vi "XYStage_Write_General_Command.vi"(5 "Timeout":i32, 7 "Command Delay":i32, 8 "error in (no error)":errorcluster, 9 "Expected Reply":string, 10 "Command to Execute":string, 11 "VISA resource name":refnum<visa-resource-name>) -> (0 "error out":errorcluster, 2 "Stage Response":string, 3 "VISA resource name out":refnum<visa-resource-name>)   [LabVIEW 2013]
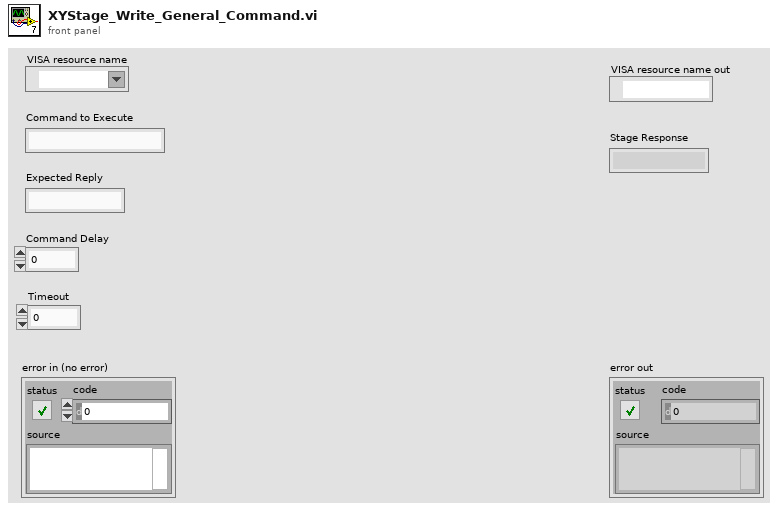
[diagram p1: front panel]
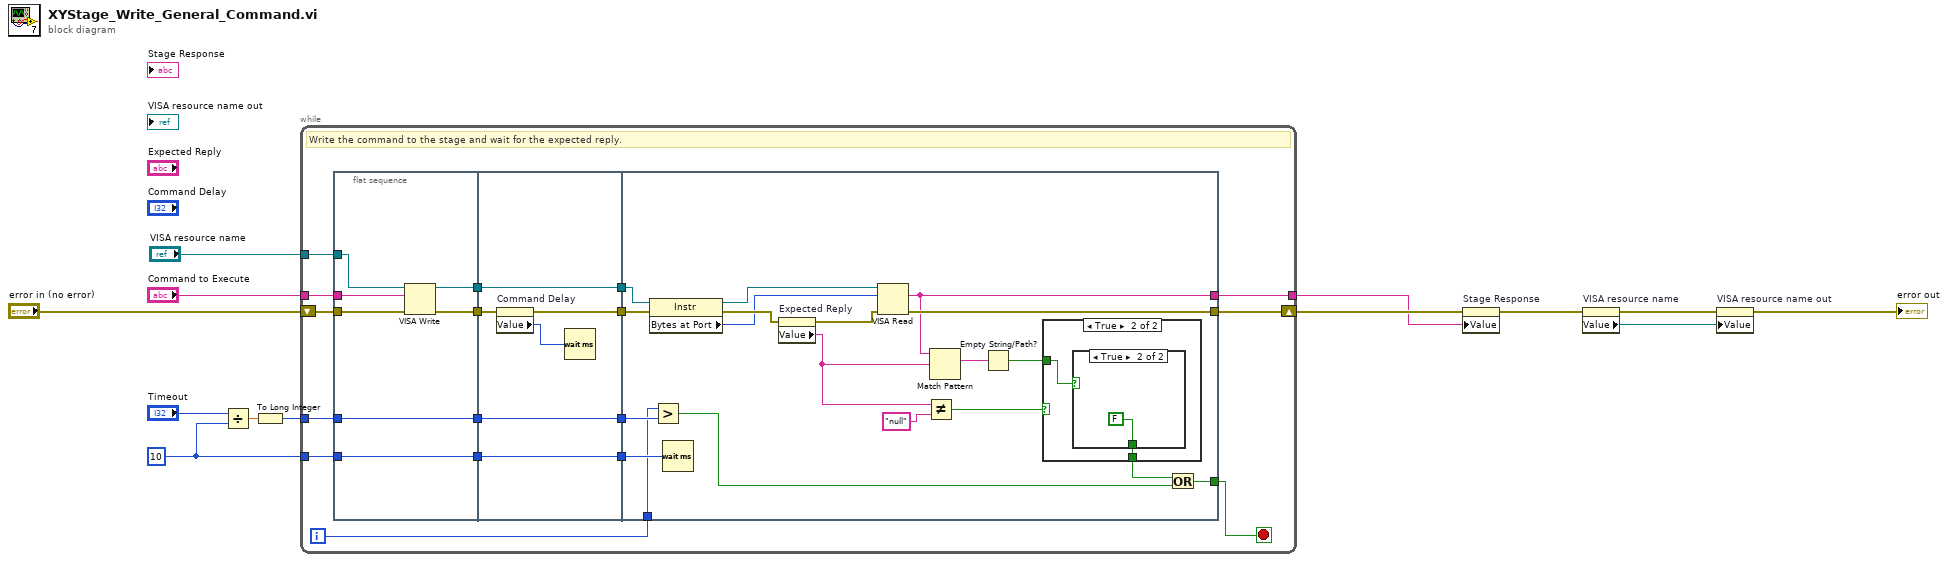
[diagram p0: block diagram]
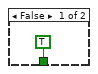
[diagram p2: hidden frame]
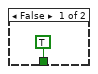
[diagram p3: hidden frame]
diagram:
  w9 = 10
  n1 = Divide(x="Timeout", y=w9) -> (x/y=w11:dbl)
  n2 = To Long Integer(number=w11) -> (32bit integer=w10:i32)
  n3 = while {
    tunnel: "VISA resource name" -> [w30]
    tunnel: "Command to Execute" -> [w29]
    shift-right: [w22] -> w6
    shift-left: "error in (no error)" -> [w28]
    tunnel: [w21] -> w5
    tunnel: w10 -> [w17]
    tunnel: w9 -> [w20]
    i -> [w14]
    stop <- w23 stop-if-true
    # "Write the command to the stage and wait for the expected reply."
    n4 = flat-sequence {
      tunnel: w30 -> [w37]
      tunnel: w29 -> [w36]
      tunnel: w28 -> [w35]
      tunnel: [w34] -> w27
      tunnel: [w33] -> w26
      tunnel: w20 -> [w32]
      tunnel: [w32] -> w19
      tunnel: w17 -> [w31]
      tunnel: [w31] -> w15
      tunnel: w27 -> [w40]
      tunnel: w26 -> [w43]
      tunnel: [w42] -> w25
      tunnel: [w40] -> w24
      tunnel: w19 -> [w39]
      tunnel: [w39] -> w18
      tunnel: [w38] -> w16
      tunnel: w15 -> [w38]
      tunnel: w25 -> [w62]
      tunnel: w24 -> [w61]
      tunnel: [w52] -> w23
      tunnel: w18 -> [w48]
      tunnel: w16 -> [w47]
      tunnel: w14 -> [w46]
      tunnel: [w50] -> w22
      tunnel: [w49] -> w21
      frame #0 {
        n5 = VISA Write(VISA resource name=w37, write buffer=w36, error in (no error)=w35) -> (VISA resource name out=w34:refnum<visa-resource-name>, error out=w33:errorcluster)  [unwired: 1 out]
      }
      frame #1 {
        n6 = property on="Command Delay" class="DigNum (strict)"(error in=w43) -> (error out=w42:errorcluster, "Value"=w41:i32)  [unwired: 1 in, 1 out]
        n7 = Wait (ms)(milliseconds to wait=w41) -> ()  [unwired: 1 out]
      }
      frame #2 {
        n8 = property class="Instr"(reference=w61, error in=w62) -> (reference out=w60:refnum<visa-resource-name>, error out=w59:errorcluster, "Bytes at Port"=w44:u32)
        n9 = Greater?(x=w46, y=w47) -> (0:w45:bool)
        n10 = Wait (ms)(milliseconds to wait=w48) -> ()  [unwired: 1 out]
        n11 = property on="Expected Reply" class="Str"(error in=w59) -> (error out=w58:errorcluster, "Value"=w57:string)  [unwired: 1 in, 1 out]
        n12 = VISA Read(VISA resource name=w60, byte count=w44, error in (no error)=w58) -> (read buffer=w49:string, error out=w50:errorcluster)  [unwired: 2 out]
        n13 = Not Equal?(x=w57, y="null") -> (x != y?=w54:bool)
        n14 = Match Pattern(string=w49, regular expression=w57) -> (match substring=w55:string)  [unwired: 1 in, 3 out]
        n15 = Empty String/Path?(string/path=w55) -> (empty?=w53:bool)
        n16 = case shown="True" w54 {
          tunnel: w53 -> [_ w65]
          tunnel: [TRUE w64] -> w51
          frame False {
          }
          frame True {
            n17 = case shown="True" w65 {
              tunnel: [TRUE FALSE] -> w64
              frame False {
              }
              frame True {
              }
            }
          }
        }
        n18 = Or(x=w51, y=w45) -> (x .or. y?=w52:bool)
      }
    }
  }
  n19 = property on="Stage Response" class="Str"(error in=w6, "Value"=w5) -> (error out=w4:errorcluster)  [unwired: 1 in, 1 out]
  n20 = property on="VISA resource name" class="VISAName"(error in=w4) -> (error out=w8:errorcluster, "Value"=w7:refnum<visa-resource-name>)  [unwired: 1 in, 1 out]
  n21 = property on="VISA resource name out" class="VISAName"(error in=w8, "Value"=w7) -> (error out=→"error out":errorcluster)  [unwired: 1 in, 1 out]
